vi "FL_Get_TTL_in_pulse_length_2.vi"(1 "Time since the last frame, s":dbl, 2 "Latest sensor input (decoded)":string[](array[string])) -> (0 "TTL pulse length, ms":u32)   [LabVIEW 2018, in "Tracker.lvlib"]
uses:
  Tracker.lvlib
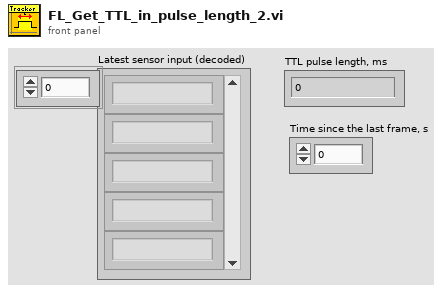
[diagram p1: front panel]
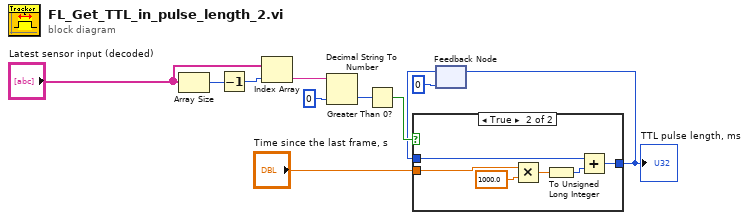
[diagram p0: block diagram]
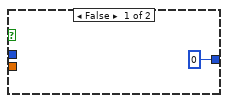
[diagram p2: hidden frame]
diagram:
  n1 = Array Size(array="Latest sensor input (decoded)") -> (size(s)=w9:i32)
  n2 = Decrement(x=w9) -> (x-1=w11:i32)
  n3 = Index Array(array="Latest sensor input (decoded)", index=w11) -> (element=w8:string)
  n4 = Decimal String To Number(string=w8, default (0L)=u8 0 ("default (0 I32)")) -> (number=w6:u8)  [unwired: 1 in, 1 out]
  n5 = Greater Than 0?(x=w6) -> (x > 0?=w5:bool)
  n6 = feedback #1(u32 0) -> (w1:u32)
  n7 = case shown="True" w5 {
    tunnel: w1 -> [_ w15]
    tunnel: "Time since the last frame, s" -> [_ w16]
    tunnel: [u32 0 w13] -> w3
    frame False {
    }
    frame True {
      n8 = Multiply(x=w16, y=1000.0) -> (x*y=w17:dbl)
      n9 = To Unsigned Long Integer(number=w17) -> (unsigned 32bit integer=w14:u32)
      n10 = Add(x=w15, y=w14) -> (x+y=w13:u32)
    }
  }
  "TTL pulse length, ms" <- w3
  n11 = feedback-in #1(w3) -> ()
